vi "mulitspot_pattern_static3_session.vi"(3 "Python error in":errorcluster, 4 "Pattern Definition":T2={"Spot pitch (pixels)"=23.1, "Tilt Angle (deg)"=0.0, "Horizontal Offset (pixels)"=91.9, "Vertical Offset (pixels)"=14.1, "# Horizontal Spots"=8, "# Vertical Spots"=1, "Spot size (pixels)"=23.1, "Darken center spot"=FALSE, "Exact Phase Formula"=TRUE, "phase wrapping"=FALSE, "Set Focus (mm)"=32.0, "Add phase"=4.0, "phase_factor"=65.0, "Steering LW"=2.0, "Steering vmax"=0.0, "phase_overshoot"=TRUE, "Focal shift param"=0.0, "x0 focal shift"=0.0, "y0 focal shift"=0.0, "hv_steering"=TRUE, "fixed"=TRUE, "Pad"=0.0, "dark_all"=FALSE, "nospot"=FALSE, "Laser wavelength"=6.28e-07} {"Laser wavelength" min=0.0 max=500.0 format="%^#.3e"; "Pad" min=0.0 max=500.0 step=1.0 format="%#.0g"; "y0 focal shift" min=0.0 max=500.0 format="%#.3g"; "x0 focal shift" min=0.0 max=500.0 format="%#.3g"; "Focal shift param" min=0.0 max=500.0 format="%#.3g"; "Steering vmax" min=0.0 max=500.0 format="%#.3g"; "Steering LW" min=0.0 max=500.0 format="%#.3g"; "phase_factor" min=0.0 max=500.0 format="%#.3f"; "Add phase" min=0.0 max=500.0 format="%#.3f"; "Set Focus (mm)" min=0.0 max=500.0 format="%#.3g"; "Spot size (pixels)" min=1.0 format="%.2g"; "# Vertical Spots" min=1 step=1; "# Horizontal Spots" min=1 step=1; "Vertical Offset (pixels)" format="%.2f"; "Horizontal Offset (pixels)" format="%.2f"; "Tilt Angle (deg)" min=-90.0 max=90.0 format="%.2g"; "Spot pitch (pixels)" min=1.0 format="%.2g"}, 5 "Python Session in":T1=refnum) -> (0 "Python error out":errorcluster, 1 "Float Matrix":dbl[][](array[numeric]), 2 "Python Session out":T1)   [LabVIEW 2011]
uses:
  Periodic Spot Pattern Parameters.ctl
  Periodic Spot Pattern Parameters2.ctl
  <userlib>/_OpenG.lib/labpython/labpython.llb/PYTHON Session Refnum__ogtk.ctl
  <userlib>/_OpenG.lib/labpython/labpython.llb/PYTHON Set Float Vector__ogtk.vi
  <userlib>/_OpenG.lib/labpython/labpython.llb/PYTHON Set Float Data__ogtk.vi
  <userlib>/_OpenG.lib/labpython/labpython.llb/PYTHON Set Integer Data__ogtk.vi
  <userlib>/_OpenG.lib/labpython/labpython.llb/PYTHON Set Boolean Data__ogtk.vi
  <userlib>/_OpenG.lib/labpython/labpython.llb/PYTHON Get Float Matrix__ogtk.vi
  <userlib>/_OpenG.lib/labpython/labpython.llb/PYTHON Get String Data__ogtk.vi
panel:
  out "Loaded script":string
  out "File error out":errorcluster
  in  "Script path":path=path "C:/Data/Antonio/software/LCOS/LCOS_CompleteLV/python/pattern_labview_session_script.py"
  in  "center_spot (to be darkened)":u16=4
  out "A string (just debug)":string="test"
  out "Xm":dbl[](array[numeric])=[21.72, 44.87, 68.2, 91.45, 114.72, 137.87, 160.97, 184.04]
  in  "Xm String (csv)":string="21.72,  44.87,  68.20,  91.45, 114.72, 137.87, 160.97, 184.04"
  out "Ym":dbl[](array[numeric])=[13.84, 13.78, 13.79, 13.83, 13.75, 13.79, 13.74, 13.68]
  in  "Ym String (csv)":string="13.84,  13.78,  13.79,  13.83,  13.75,  13.79,  13.74,  13.68"
  out "Intensity Graph":dbl[][](graph)
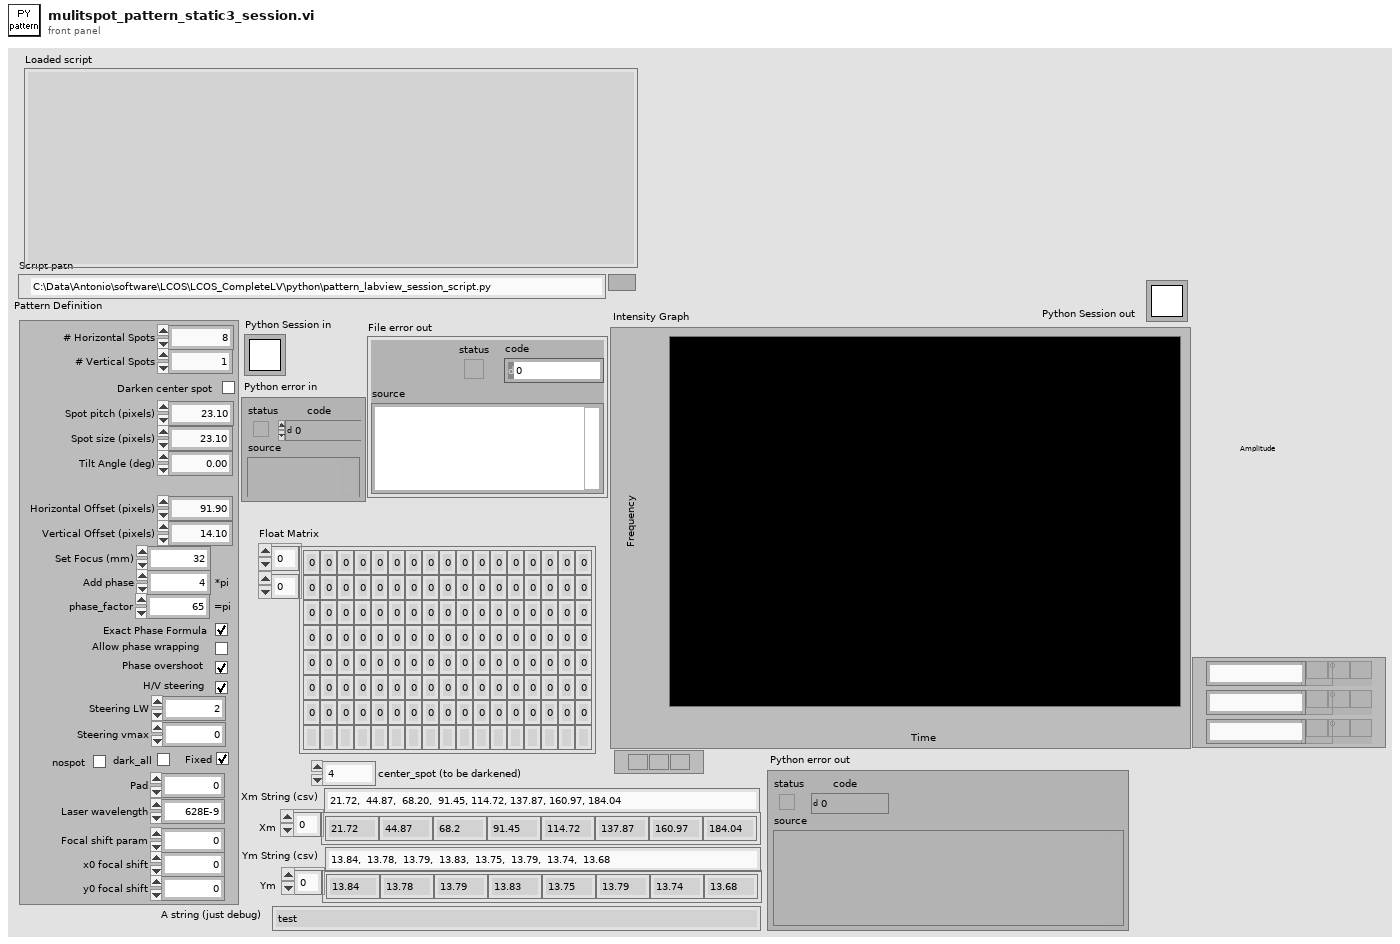
[diagram p1: front panel]
types:
  T1 = typedef "PYTHON Session Refnum__ogtk.ctl" = refnum<k1>
  T2 = typedef "Periodic Spot Pattern Parameters.ctl" = cluster{"Spot pitch (pixels)":dbl, "Tilt Angle (deg)":dbl, "Horizontal Offset (pixels)":dbl, "Vertical Offset (pixels)":dbl, "# Horizontal Spots":u32, "# Vertical Spots":u32, "Spot size (pixels)":dbl, "Darken center spot":bool, "Exact Phase Formula":bool, "phase wrapping":bool, "Set Focus (mm)":T3, "Add phase":dbl, "phase_factor":dbl, "Steering LW":T3, "Steering vmax":T3, "phase_overshoot":bool, "Focal shift param":T3, "x0 focal shift":T3, "y0 focal shift":T3, "hv_steering":bool, "fixed":bool, "Pad":T3, "dark_all":bool, "nospot":bool, "Laser wavelength":dbl}
  T3 = typedef "Periodic Spot Pattern Parameters2.ctl" = dbl
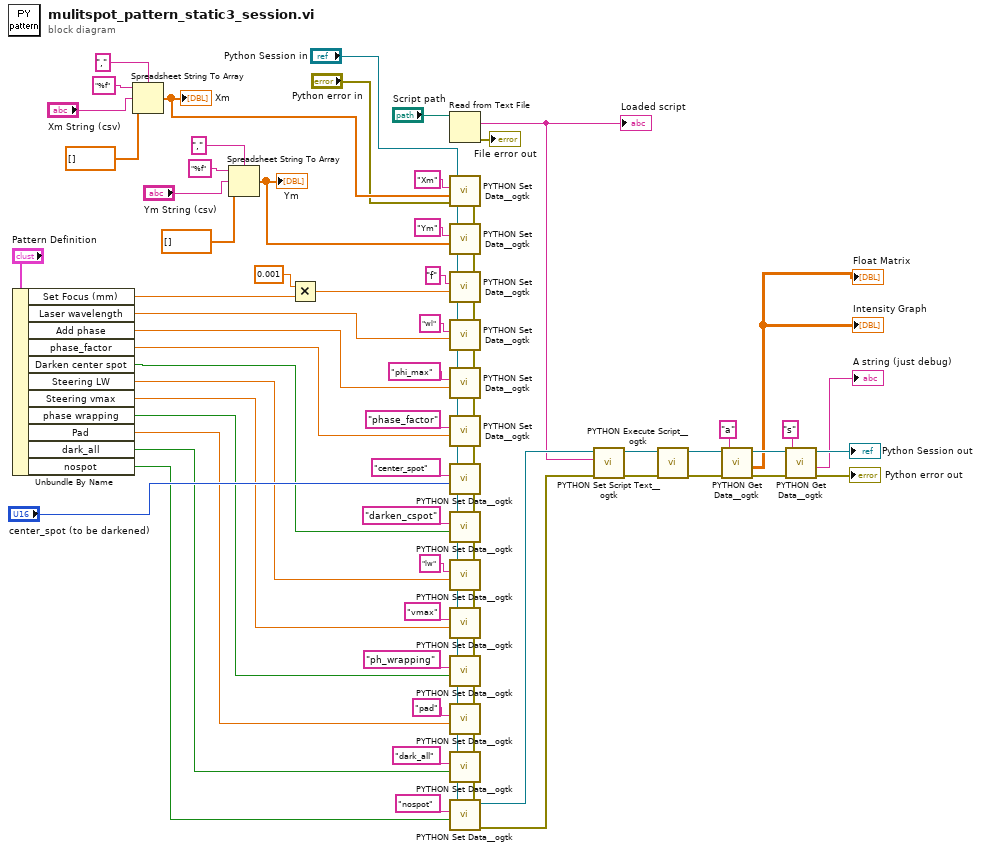
[diagram p0: block diagram]
diagram:
  n1 = Unbundle By Name("Pattern Definition") -> ("Set Focus (mm)"=w75:T3, "Laser wavelength"=w30:dbl, "Add phase"=w29:dbl, "phase_factor"=w28:dbl, "Darken center spot"=w26:bool, "Steering LW"=w25:T3, "Steering vmax"=w24:T3, "phase wrapping"=w23:bool, "Pad"=w22:T3, "dark_all"=w21:bool, "nospot"=w20:bool)
  n2 = Spreadsheet String To Array(delimiter (Tab)=",", format string="%f", spreadsheet string="Xm String (csv)", array type (2D Dbl)=dbl[] []) -> (array=w33:dbl[])
  "Xm" <- w33
  n3 = Spreadsheet String To Array(delimiter (Tab)=",", format string="%f", spreadsheet string="Ym String (csv)", array type (2D Dbl)=dbl[] []) -> (array=w32:dbl[])
  "Ym" <- w32
  n4 = Multiply(x=T3 0.001, y=w75) -> (x*y=w31:T3)
  n5 = Read from Text File(file (use dialog)="Script path") -> (text=w10:string, error out=→"File error out":errorcluster)  [unwired: 3 in, 2 out]
  "Loaded script" <- w10
  n6 = call-poly <userlib>:"PYTHON Set Data__ogtk.vi"("error in (no error)"="Python error in", "value"=w33, "variable name"="Xm", "Python Session in"="Python Session in") -> ("error out"=w62:errorcluster, "Python Session out"=w73:T1)  [unwired: 2 in]
  n7 = call-poly <userlib>:"PYTHON Set Data__ogtk.vi"("error in (no error)"=w62, "value"=w32, "variable name"="Ym", "Python Session in"=w73) -> ("error out"=w61:errorcluster, "Python Session out"=w72:T1)  [unwired: 2 in]
  n8 = call-poly <userlib>:"PYTHON Set Data__ogtk.vi"("error in (no error)"=w61, "value"=w31, "variable name"="f", "Python Session in"=w72) -> ("error out"=w60:errorcluster, "Python Session out"=w71:T1)  [unwired: 2 in]
  n9 = call-poly <userlib>:"PYTHON Set Data__ogtk.vi"("error in (no error)"=w60, "value"=w30, "variable name"="wl", "Python Session in"=w71) -> ("error out"=w59:errorcluster, "Python Session out"=w70:T1)  [unwired: 2 in]
  n10 = call-poly <userlib>:"PYTHON Set Data__ogtk.vi"("error in (no error)"=w59, "value"=w29, "variable name"="phi_max", "Python Session in"=w70) -> ("error out"=w58:errorcluster, "Python Session out"=w69:T1)  [unwired: 2 in]
  n11 = call-poly <userlib>:"PYTHON Set Data__ogtk.vi"("error in (no error)"=w58, "value"=w28, "variable name"="phase_factor", "Python Session in"=w69) -> ("error out"=w57:errorcluster, "Python Session out"=w68:T1)  [unwired: 2 in]
  n12 = call-poly <userlib>:"PYTHON Set Data__ogtk.vi"("error in (no error)"=w57, "value"="center_spot (to be darkened)", "variable name"="center_spot", "Python Session in"=w68) -> ("error out"=w56:errorcluster, "Python Session out"=w67:T1)  [unwired: 2 in]
  n13 = call-poly <userlib>:"PYTHON Set Data__ogtk.vi"("error in (no error)"=w56, "value"=w26, "variable name"="darken_cspot", "Python Session in"=w67) -> ("error out"=w55:errorcluster, "Python Session out"=w66:T1)  [unwired: 2 in]
  n14 = call-poly <userlib>:"PYTHON Set Data__ogtk.vi"("error in (no error)"=w55, "value"=w25, "variable name"="lw", "Python Session in"=w66) -> ("error out"=w54:errorcluster, "Python Session out"=w65:T1)  [unwired: 2 in]
  n15 = call-poly <userlib>:"PYTHON Set Data__ogtk.vi"("error in (no error)"=w54, "value"=w24, "variable name"="vmax", "Python Session in"=w65) -> ("error out"=w53:errorcluster, "Python Session out"=w64:T1)  [unwired: 2 in]
  n16 = call-poly <userlib>:"PYTHON Set Data__ogtk.vi"("error in (no error)"=w53, "value"=w23, "variable name"="ph_wrapping", "Python Session in"=w64) -> ("error out"=w38:errorcluster, "Python Session out"=w63:T1)  [unwired: 2 in]
  n17 = call-poly <userlib>:"PYTHON Set Data__ogtk.vi"("error in (no error)"=w38, "value"=w22, "variable name"="pad", "Python Session in"=w63) -> ("error out"=w37:errorcluster, "Python Session out"=w35:T1)  [unwired: 2 in]
  n18 = call-poly <userlib>:"PYTHON Set Data__ogtk.vi"("error in (no error)"=w37, "value"=w21, "variable name"="dark_all", "Python Session in"=w35) -> ("error out"=w36:errorcluster, "Python Session out"=w34:T1)  [unwired: 2 in]
  n19 = call-poly <userlib>:"PYTHON Set Data__ogtk.vi"("error in (no error)"=w36, "value"=w20, "variable name"="nospot", "Python Session in"=w34) -> ("error out"=w15:errorcluster, "Python Session out"=w19:T1)  [unwired: 2 in]
  n20 = call <userlib>:"PYTHON Set Script Text__ogtk.vi"("error in (no error)"=w15, "script text"=w10, "Python Session in"=w19) -> ("error out"=w14:errorcluster, "Python Session out"=w18:T1)  [unwired: 3 in]
  n21 = call <userlib>:"PYTHON Execute Script__ogtk.vi"("error in (no error)"=w14, "Python Session in"=w18) -> ("error out"=w13:errorcluster, "Python Session out"=w17:T1)  [unwired: 4 in]
  n22 = call-poly <userlib>:"PYTHON Get Data__ogtk.vi"("error in (no error)"=w13, "variable name"="a", "Python Session in"=w17) -> ("error out"=w12:errorcluster, "value"=→"Float Matrix" →"Intensity Graph":dbl[][], "Python Session out"=w16:T1)  [unwired: 2 in]
  n23 = call-poly <userlib>:"PYTHON Get Data__ogtk.vi"("error in (no error)"=w12, "variable name"="s", "Python Session in"=w16) -> ("error out"=→"Python error out":errorcluster, "value"=→"A string (just debug)":string, "Python Session out"=→"Python Session out":T1)  [unwired: 2 in]
